vi "Initialize Dependency.vi"(6 "Shared Resource (T)":bool, 7 "Dependency":refnum<class "Dependency.lvclass">, 8 "error in (no error)":errorcluster, 9 "Start Order (0)":i8, 10 "Name":string, 11 "Type":refnum<class "SMO.lvclass">) -> (0 "error out":errorcluster, 3 "Dependency out":refnum<class "Dependency.lvclass">)   [LabVIEW 2013, in "Dependency.lvclass"]
uses:
  Dependency.lvclass
  SMO/SMO.lvclass
  Dependency.lvclass/Dependency.ctl
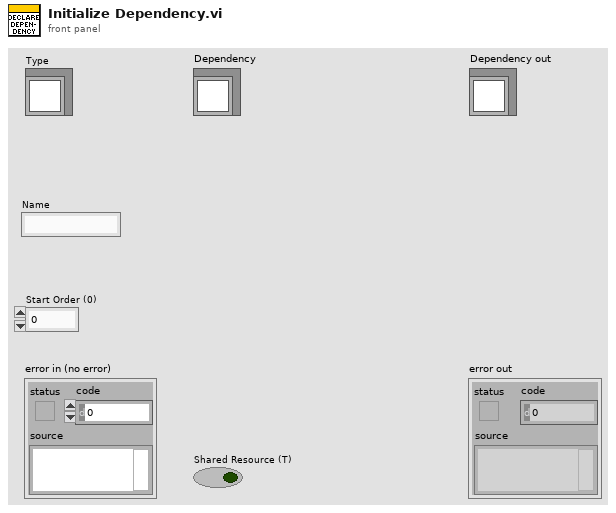
[diagram p1: front panel]
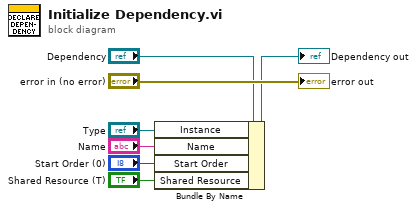
[diagram p0: block diagram]
diagram:
  n1 = Bundle By Name(cluster="Dependency", "Instance"="Type", "Name"="Name", "Start Order"="Start Order (0)", "Shared Resource"="Shared Resource (T)") -> (→"Dependency out":refnum<class "Dependency.lvclass">)
  "error out" <- "error in (no error)"
